vi "Play Async Invoke.vi"() -> ()   [LabVIEW 2018]
uses:
  TwinCAT ADS Class/VIs/Data/Invoke Method.vi
  TwinCAT ADS Class/VIs/Data/Read.vi
  TwinCAT ADS Class/TwinCAT ADS.lvclass
panel:
  in  "Read":bool
  in  "Stop":bool
  in  "Invoke":bool
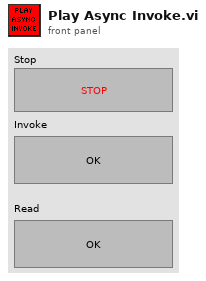
[diagram p1: front panel]
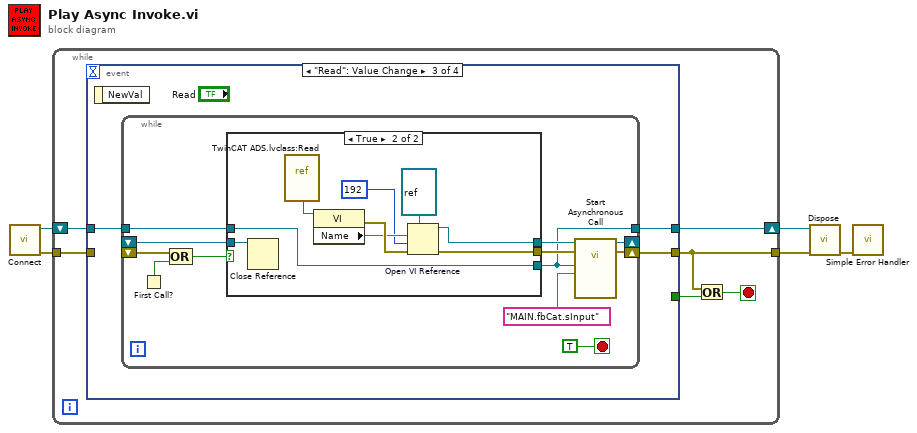
[diagram p0: block diagram]
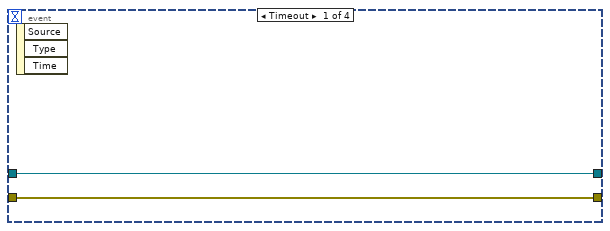
[diagram p2: hidden frame]
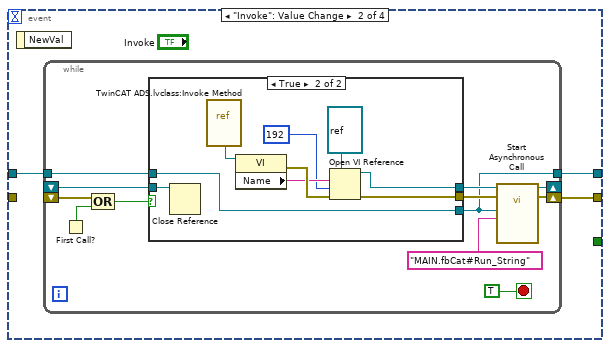
[diagram p3: hidden frame]
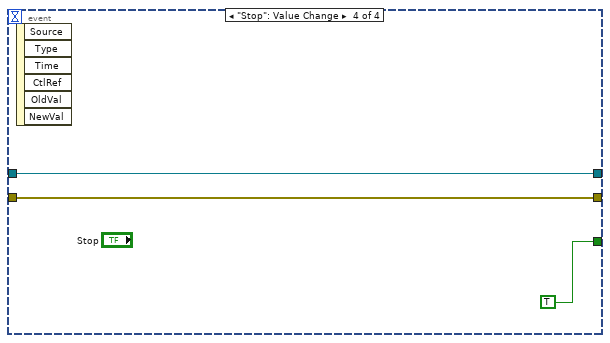
[diagram p6: hidden frame]
diagram:
  n1 = call "Connect.vi"() -> ("error out"=w4:errorcluster, "TwinCAT ADS out"=w5:refnum<class "TwinCAT ADS.lvclass">)  [unwired: 10 in]
  n2 = while {
    shift-right: [w9] -> w3
    shift-left: w5 -> [w11]
    tunnel: w4 -> [w10]
    tunnel: [w8] -> w2
    stop <- w6 stop-if-true
    n3 = event shown="[2] \"Read\": Value Change" {
      selector: _ -> [_ _ _ _]
      dyn-events: _ -> [_ _ _ _]
      timeout: _ -> [_ _ _ _]
      tunnel: [_ _ _ TRUE] -> w7
      tunnel: w11 -> [w13 w16 w42 w67]
      tunnel: w10 -> [w12 _ _ w66]
      tunnel: [w13 w14 w40 w67] -> w9
      tunnel: [w12 w15 w41 w66] -> w8
      event Timeout {
        n4 = event-data() -> ()  [unwired: 1 in, 3 out]
      }
      event "Invoke": Value Change {
        n5 = event-data() -> ()  [unwired: 1 in, 1 out]
        n6 = while {
          tunnel: w16 -> [w19]
          shift-right: [w27] -> w15
          shift-left: _ -> [w24]
          shift-right: [w26] -> _
          shift-left: _ -> [w25]
          tunnel: [w17] -> w14
          stop <- TRUE stop-if-true
          n7 = First Call?() -> (First Call?: T/F=w23:bool)
          n8 = Compound Arithmetic op=OR(w24, w23) -> (w22:bool)
          n9 = case shown="True" w22 {
            tunnel: w25 -> [w30 w36]
            tunnel: [_ w39] -> w21
            tunnel: [w30 w38] -> w20
            tunnel: w19 -> [w29 w32]
            tunnel: [w29 w32] -> w17
            frame False {
            }
            frame True {
              n10 = Close Reference(reference=w36) -> ()  [unwired: 1 in, 1 out]
              n11 = vi-ref "TwinCAT ADS.lvclass:Invoke Method.vi"() -> (w35:refnum<vi>)
              n12 = property class="VI"(reference=w35) -> (error out=w34:errorcluster, "Name"=w33:string)  [unwired: 1 in, 1 out]
              n13 = Open VI Reference(type specifier VI Refnum (for type only)=refnum<vi> refnum, vi path=w33, options=192, error in (no error)=w34) -> (vi reference=w38:refnum<vi>, error out=w39:errorcluster)  [unwired: 2 in]
            }
          }
          n14 = call-by-ref "Start Asynchronous Call"(reference=w20, error in=w21, "Function Block/Program#Method"="MAIN.fbCat#Run_String", "TwinCAT ADS in"=w17) -> (reference out=w26:refnum<vi>, error out=w27:errorcluster)  [unwired: 6 in, 4 out]
        }
      }
      event "Read": Value Change {
        n15 = event-data() -> ()  [unwired: 1 in, 1 out]
        n16 = while {
          tunnel: w42 -> [w45]
          shift-right: [w53] -> w41
          shift-left: _ -> [w50]
          shift-right: [w52] -> _
          shift-left: _ -> [w51]
          tunnel: [w43] -> w40
          stop <- TRUE stop-if-true
          n17 = First Call?() -> (First Call?: T/F=w49:bool)
          n18 = Compound Arithmetic op=OR(w50, w49) -> (w48:bool)
          n19 = case shown="True" w48 {
            tunnel: w51 -> [w56 w63]
            tunnel: [_ w65] -> w47
            tunnel: [w56 w64] -> w46
            tunnel: w45 -> [w55 w59]
            tunnel: [w55 w59] -> w43
            frame False {
            }
            frame True {
              n20 = Close Reference(reference=w63) -> ()  [unwired: 1 in, 1 out]
              n21 = vi-ref "TwinCAT ADS.lvclass:Read.vi"() -> (w62:refnum<vi>)
              n22 = property class="VI"(reference=w62) -> (error out=w61:errorcluster, "Name"=w60:string)  [unwired: 1 in, 1 out]
              n23 = Open VI Reference(type specifier VI Refnum (for type only)=refnum<vi> refnum, vi path=w60, options=192, error in (no error)=w61) -> (vi reference=w64:refnum<vi>, error out=w65:errorcluster)  [unwired: 2 in]
            }
          }
          n24 = call-by-ref "Start Asynchronous Call"(reference=w46, error in=w47, "Symbol Name"="MAIN.fbCat.sInput" ("Function Block/Program#Method"), "TwinCAT ADS in"=w43) -> (reference out=w52:refnum<vi>, error out=w53:errorcluster)  [unwired: 7 in, 3 out]
        }
      }
      event "Stop": Value Change {
        n25 = event-data() -> ()  [unwired: 1 in, 6 out]
      }
    }
    n26 = Or(x=w8, y=w7) -> (x .or. y?=w6:bool)
  }
  n27 = call "Dispose.vi"("error in (no error)"=w2, "TwinCAT ADS in"=w3) -> ("error out"=w1:errorcluster)  [unwired: 9 in]
  n28 = call <vilib>:"Simple Error Handler.vi"("error in (no error)"=w1) -> ()  [unwired: 4 in, 5 out]
